vi "List2.vi"() -> ()   [LabVIEW 2017]
uses:
  <vilib>/Instr/_visa.llb/VISA Configure Serial Port (Instr).vi
panel:
  out "Waveform Chart":dbl(graph)
  out "Wynik":string
  in  "Tryb":bool
  out "Wartoœæ poza zakresem miernika":bool
  out "Temperatura poza zakresem czunika":bool
  in  "Skala":bool
  in  "Precyzja":u8
  in  "Rodzaj czujnika":u8(knob) scale=0.0..1.0
  out "B酬dy komunikacji":errorcluster
  in  "Delay [ms]":dbl=500.0 min=500.0 max=10000.0 step=1.0
  in  "Stop":bool
  # "oC"
  # "Rezytancja"
  # "oF"
  # "Temperatura"
  # "BＪDY"
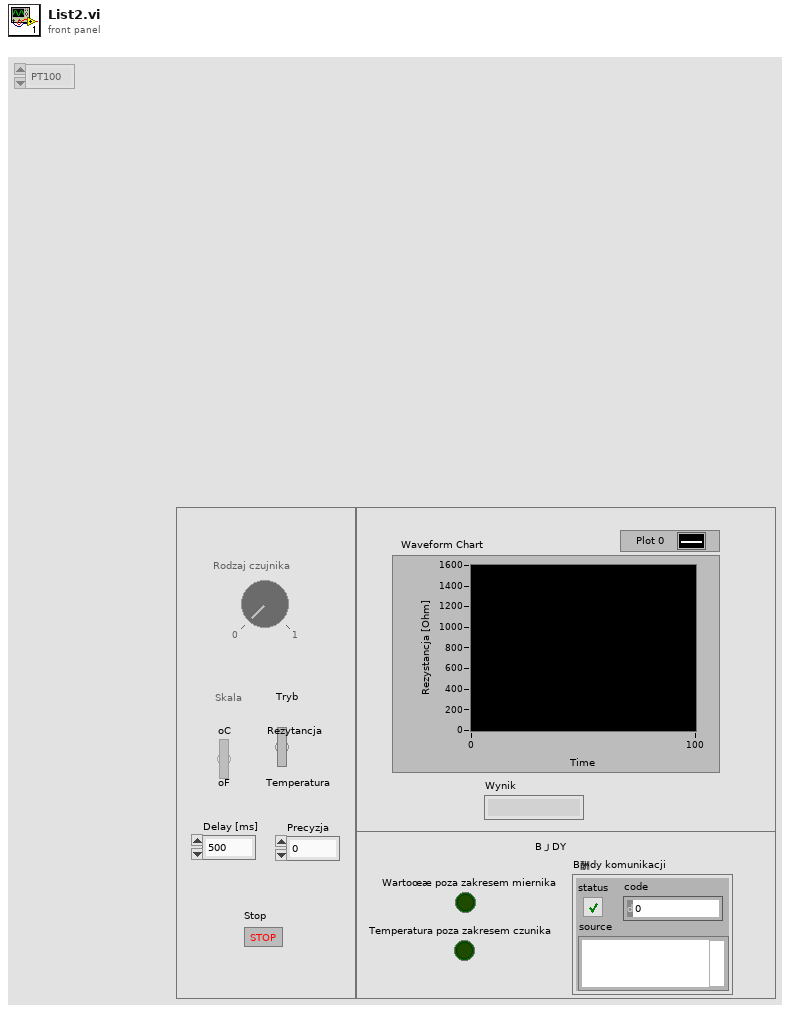
[diagram p1: front panel]
types:
  T1 = enum8{"Enabled", "Disabled", "Disabled and Grayed Out"}
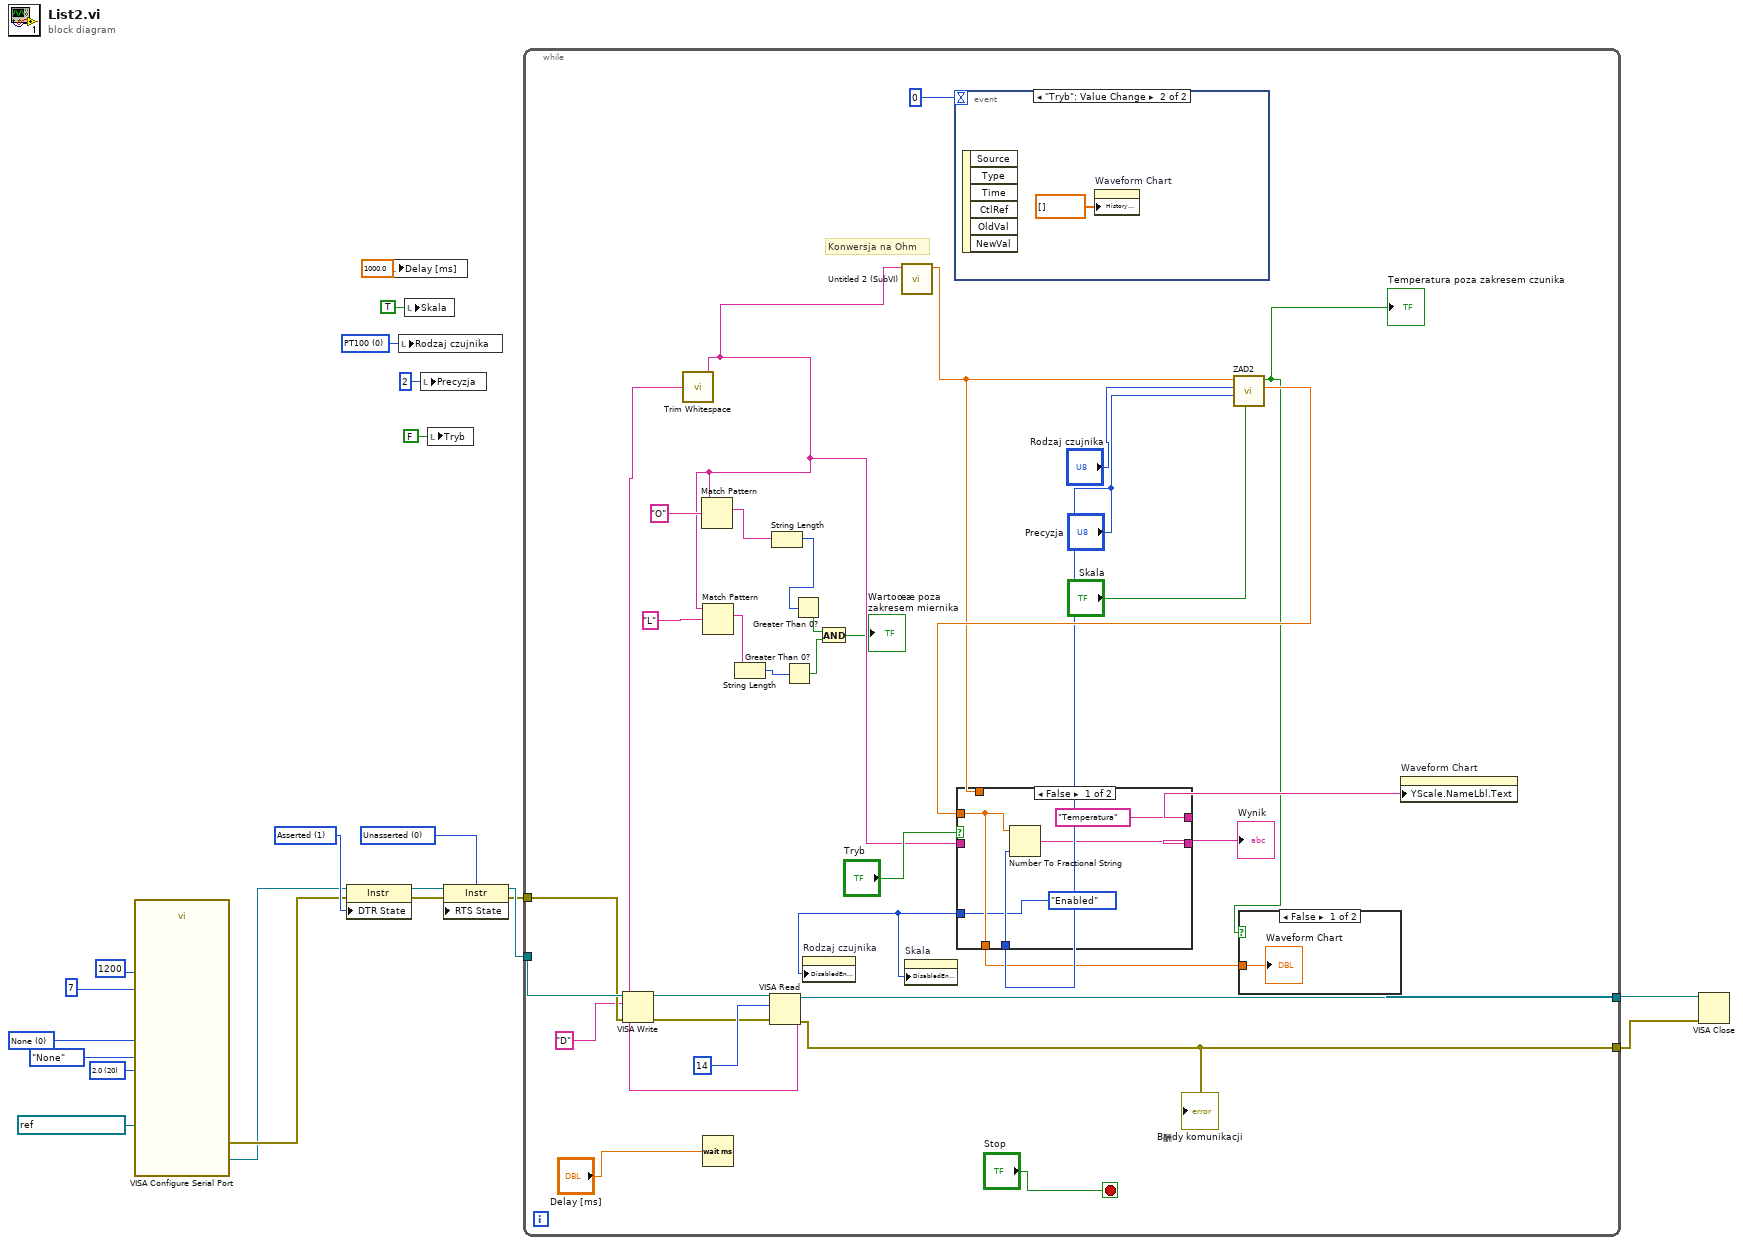
[diagram p0: block diagram]
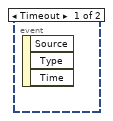
[diagram p3: hidden frame]
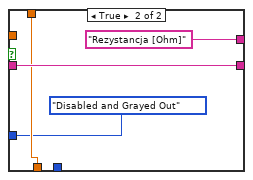
[diagram p4: hidden frame]
diagram:
  w4 = 0 items=["PT100", "KTY81-210"] ("Rodzaj czujnika")
  w14 = i16 0 items=["Unknown"=-1, "Unasserted"=0, "Asserted"=1] ("Serial Settings:Modem Line Settings:Line RTS State")
  w15 = i16 1 items=["Unknown"=-1, "Unasserted"=0, "Asserted"=1] ("Serial Settings:Modem Line Settings:Line DTR State")
  w17 = u16 0 items=["None", "XON/XOFF", "RTS/CTS", "XON/XOFF & RTS/CTS", "DTR/DSR", "XON/XOFF & DTR/DSR"] ("flow control (0:none)")
  w19 = u16 20 items=["1.0"=10, "1.5"=15, "2.0"=20] ("stop bits (10: 1 bit)")
  n1 = call-poly "VISA Configure Serial Port"("VISA resource name"=refnum<visa-resource-name> "COM1", "baud rate (9600)"=u32 1200, "data bits (8)"=u16 7, "parity (0:none)"=enum16{"None", "Odd", "Even", "Mark", "Space"}."None", "stop bits (10: 1 bit)"=w19, "flow control (0:none)"=w17) -> ("VISA resource name out"=w12:refnum<visa-resource-name>, "error out"=w13:errorcluster)  [unwired: 8 in]
  n2 = property class="Instr"(reference=w12, error in=w13, "DTR State"=w15) -> (reference out=w10:refnum<visa-resource-name>, error out=w11:errorcluster)
  n3 = local write "Delay [ms]"(1000.0 ("Delay")) -> ()
  n4 = local write "Rodzaj czujnika"(w4) -> ()
  n5 = local write "Skala"(TRUE ("Skala")) -> ()
  n6 = local write "Precyzja"(2 ("Precyzja")) -> ()
  n7 = local write "Tryb"(FALSE ("Tryb")) -> ()
  n8 = property class="Instr"(reference=w10, error in=w11, "RTS State"=w14) -> (reference out=w9:refnum<visa-resource-name>, error out=w8:errorcluster)
  n9 = while {
    tunnel: w9 -> [w53]
    tunnel: w8 -> [w52]
    tunnel: [w47] -> w1
    tunnel: [w46] -> w6
    stop <- "Stop" stop-if-true
    # "Konwersja na Ohm"
    n10 = VISA Write(VISA resource name=w53, write buffer="D", error in (no error)=w52) -> (VISA resource name out=w49:refnum<visa-resource-name>, error out=w48:errorcluster)  [unwired: 1 out]
    n11 = Wait (ms)(milliseconds to wait="Delay [ms]") -> ()  [unwired: 1 out]
    n12 = VISA Read(VISA resource name=w49, byte count=u32 14, error in (no error)=w48) -> (VISA resource name out=w46:refnum<visa-resource-name>, read buffer=w43:string, error out=w47:errorcluster)  [unwired: 1 out]
    "B酬dy komunikacji" <- w47
    n13 = call <vilib>:"Trim Whitespace.vi"("string"=w43) -> ("trimmed string"=w28:string)  [unwired: 1 in]
    n14 = Match Pattern(string=w28, regular expression="O") -> (match substring=w41:string)  [unwired: 1 in, 3 out]
    n15 = Match Pattern(string=w28, regular expression="L") -> (match substring=w26:string)  [unwired: 1 in, 3 out]
    n16 = String Length(string=w26) -> (length=w25:i32)
    n17 = String Length(string=w41) -> (length=w40:i32)
    n18 = Greater Than 0?(x=w25) -> (x > 0?=w24:bool)
    n19 = Greater Than 0?(x=w40) -> (x > 0?=w23:bool)
    n20 = And(x=w23, y=w24) -> (x .and. y?=→"Wartoœæ poza zakresem miernika":bool)
    n21 = call "Untitled 2 (SubVI).vi"("trimmed string"=w28) -> ("Numeric"=w35:dbl)  [unwired: 10 in]
    n22 = event shown="[1] \"Tryb\": Value Change" {
      selector: _ -> [_ _]
      dyn-events: _ -> [_ _]
      timeout: 0 -> [_ _]
      event Timeout {
        n23 = event-data() -> ()  [unwired: 1 in, 3 out]
      }
      event "Tryb": Value Change {
        n24 = event-data() -> ()  [unwired: 1 in, 6 out]
        n25 = property on="Waveform Chart" class="WFChart (strict)"("History Data"=dbl[] []) -> ()  [unwired: 2 in, 2 out]
      }
    }
    n26 = call "ZAD2.vi"("Skala"="Skala", "Precyzja"="Precyzja", "Rodzaj czujnika"="Rodzaj czujnika", "Numeric in"=w35) -> ("Numeric out"=w39:dbl, "Error"=w31:bool)  [unwired: 6 in]
    "Temperatura poza zakresem czunika" <- w31
    n27 = case shown="False" "Tryb" {
      tunnel: w39 -> [w58 _]
      tunnel: [w61 w65] -> w37
      tunnel: w28 -> [_ w65]
      tunnel: "Precyzja" -> [w60 _]
      tunnel: w35 -> [_ w63]
      tunnel: ["Temperatura" ("Y Scale.Name Label.Text") "Rezystancja [Ohm]" ("Y Scale.Name Label.Text")] -> w34
      tunnel: [w58 w63] -> w30
      tunnel: [T1."Enabled" ("Disabled") T1."Disabled and Grayed Out" ("Disabled")] -> w29
      frame False {
        n28 = Number To Fractional String(number=w58, precision (6)=w60) -> (F-format string=w61:string)  [unwired: 2 in]
      }
      frame True {
      }
    }
    "Wynik" <- w37
    n29 = property on="Rodzaj czujnika" class="Knob (strict)"("DisabledEnum"=w29) -> ()  [unwired: 2 in, 2 out]
    n30 = property on="Skala" class="Bool (strict)"("DisabledEnum"=w29) -> ()  [unwired: 2 in, 2 out]
    n31 = case shown="False" w31 {
      tunnel: w30 -> [w55 _]
      frame False {
        "Waveform Chart" <- w55
      }
      frame True {
      }
    }
    n32 = property on="Waveform Chart" class="WFChart (strict)"("YScale.NameLbl.Text"=w34) -> ()  [unwired: 2 in, 2 out]
  }
  n33 = VISA Close(VISA resource name=w6, error in (no error)=w1) -> ()  [unwired: 1 out]
